vi "Pass_parameters_to_card_control.vi"(8 "error in (no error)":errorcluster, 10 "Control_card.lvclass":refnum<class "Control_card.lvclass">, 11 "Control_interface in":refnum<class "Control_interface.lvclass">) -> (0 "error out":errorcluster, 2 "Initialize_card out":refnum<class "Control_card.lvclass">, 3 "Control_interface out":refnum<class "Control_interface.lvclass">)   [LabVIEW 2015, in "Control_interface.lvclass"]
uses:
  Control_interface.lvclass
  Control_card.lvclass
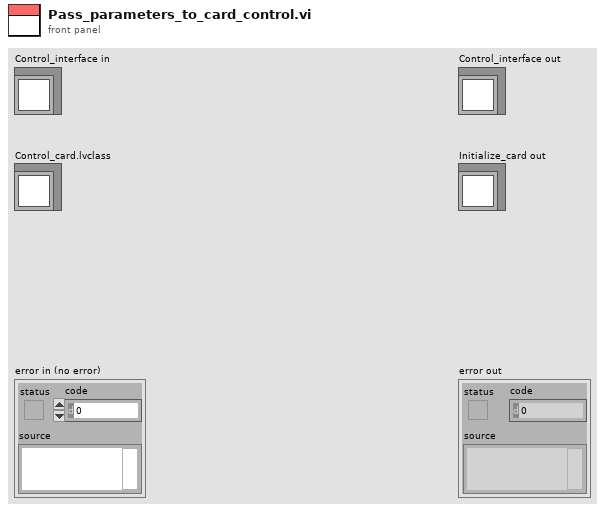
[diagram p1: front panel]
types:
  T1 = cluster{"Sample Rate":dbl, "Clock mode":enum16{"Internal", "External", "Reference"}, "Mode":u16, "Depth":dbl, "Segment Size":dbl, "Trigger Timeout":dbl, "Trigger Holdoff":dbl, "Trigger Delay":dbl}
  T2 = cluster{"Coupling":u16, "Differential Input":bool, "Direct-to-ADC":bool, "Range":u32, "Impedance":u32, "DC Offset":i32, "Filter":i32}
  T3 = cluster{"Slope":u16, "Level":i32, "Source":i32, "External Range":u32, "External Coupling":u16, "External":bool, "Disable":bool, "External Impedance":u16}
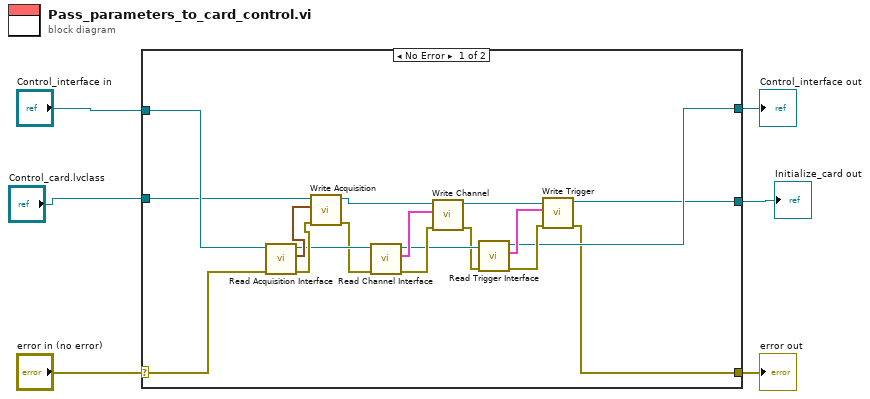
[diagram p0: block diagram]
diagram:
  n1 = case shown="No Error" "error in (no error)" {
    selector: "error in (no error)" -> [w10 w27]
    tunnel: [w9 w27] -> w5
    tunnel: [w11 w26] -> w3
    tunnel: "Control_interface in" -> [w12 w26]
    tunnel: "Control_card.lvclass" -> [w8 w25]
    tunnel: [w7 w25] -> w1
    frame No Error {
      n2 = call-dynamic "Read Acquisition Interface.vi"("error in (no error)"=w10, "Control_interface in"=w12) -> ("error out"=w23:errorcluster, "Acquisition Interface"=w24:T1, "Control_interface out"=w22:refnum<class "Control_interface.lvclass">)  [unwired: 7 in]
      n3 = call-dynamic "Write Acquisition.vi"("error in (no error)"=w23, "Acquisition"=w24, "Initialize_card in"=w8) -> ("error out"=w21:errorcluster, "Initialize_card out"=w20:refnum<class "Control_card.lvclass">)  [unwired: 7 in]
      n4 = call-dynamic "Read Channel Interface.vi"("error in (no error)"=w21, "Control_interface in"=w22) -> ("error out"=w18:errorcluster, "Channel Interface"=w19:T2, "Control_interface out"=w17:refnum<class "Control_interface.lvclass">)  [unwired: 7 in]
      n5 = call-dynamic "Write Channel.vi"("error in (no error)"=w18, "Channel"=w19, "Initialize_card in"=w20) -> ("error out"=w16:errorcluster, "Initialize_card out"=w15:refnum<class "Control_card.lvclass">)  [unwired: 7 in]
      n6 = call-dynamic "Read Trigger Interface.vi"("error in (no error)"=w16, "Control_interface in"=w17) -> ("error out"=w13:errorcluster, "Trigger Interface"=w14:T3, "Control_interface out"=w11:refnum<class "Control_interface.lvclass">)  [unwired: 7 in]
      n7 = call-dynamic "Write Trigger.vi"("error in (no error)"=w13, "Trigger"=w14, "Initialize_card in"=w15) -> ("error out"=w9:errorcluster, "Initialize_card out"=w7:refnum<class "Control_card.lvclass">)  [unwired: 7 in]
    }
    frame Error {
    }
  }
  "error out" <- w5
  "Control_interface out" <- w3
  "Initialize_card out" <- w1
